vi "Get Item Name.vi"(8 "error in":errorcluster, 11 "item ref in":T1 format="%.0x") -> (0 "error out":errorcluster, 2 "name":string, 3 "item ref out":T1 format="%.0x")   [LabVIEW 2020, in "Custom Device Serialization.lvlib"]
uses:
  Custom Device Serialization.lvlib
  <vilib>/NI VeriStand/Custom Device API/Custom Device API.lvlib
  <vilib>/NI VeriStand/Custom Device API/Custom Device Item Ref.ctl
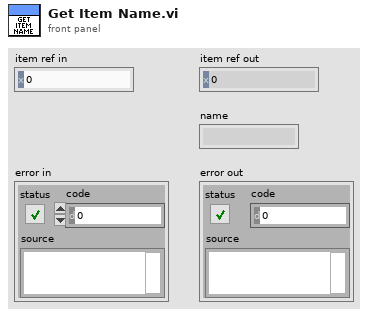
[diagram p1: front panel]
types:
  T1 = typedef "Custom Device API.lvlib/Custom Device Item Ref.ctl" = u64
  T2 = typedef "Custom Device API.lvlib/Custom Device Item Info.ctl" = cluster{"Name":string, "Is Channel":bool, "GUID":string, "Is Waveform":bool}
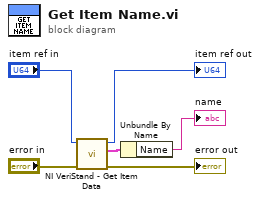
[diagram p0: block diagram]
diagram:
  n1 = call <vilib>:"NI VeriStand - Get Item Data.vi"("error in (no error)"="error in", "Item Ref in"="item ref in") -> ("error out"=→"error out":errorcluster, "Item Info"=w3:T2, "Item Ref out"=→"item ref out":T1)  [unwired: 6 in, 1 out]
  n2 = Unbundle By Name(w3) -> ("Name"=→"name":string)
